vi "WebDAV Credentials.vi"() -> (2 "Password":string, 3 "Username":string="admin")   [LabVIEW 2021, in "BS120x Driver.lvlib" / "ENET_BS1200.lvclass"]
uses:
  ENET_BS1200.lvclass
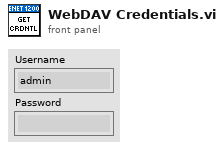
[diagram p1: front panel]
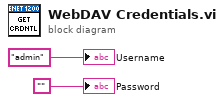
[diagram p0: block diagram]
diagram:
  "Username" <- "admin"
  "Password" <- ""
